vi "Speciality IO Channel Names.vi"(8 "error in (no error)":errorcluster, 10 "channel in":T1, 11 "FPGA Addon ref in":T3 format="%.0x") -> (0 "error out":errorcluster, 2 "channel names out":string[](array[string]), 3 "FPGA Addon ref out":T3 format="%.0x")   [LabVIEW 2026, in "FPGA Addon Bitfile Reload Unit Tests.lvclass"]
uses:
  FPGA Addon Bitfile Reload Unit Tests.lvclass
  <vilib>/NI VeriStand/Custom Device API/Custom Device API.lvlib
  <vilib>/NI VeriStand/Custom Device Tools/Custom Device Utility Library/Custom Device Utility Library.lvlib
  <vilib>/NI VeriStand/Custom Device Tools/Custom Device Utility Library/NI VeriStand - Search for Item by Name.vi
  <vilib>/NI VeriStand/Custom Device API/Custom Device Item Ref.ctl
  APIs/Scripting API/TypeDefs/Output Scalar Data.ctl
  APIs/Scripting API/Scripting API.lvlib
  Addon/Addon Shared/Types/FPGA Addon Data Type.ctl
  Addon/Addon Shared/FPGA Addon Shared.lvlib
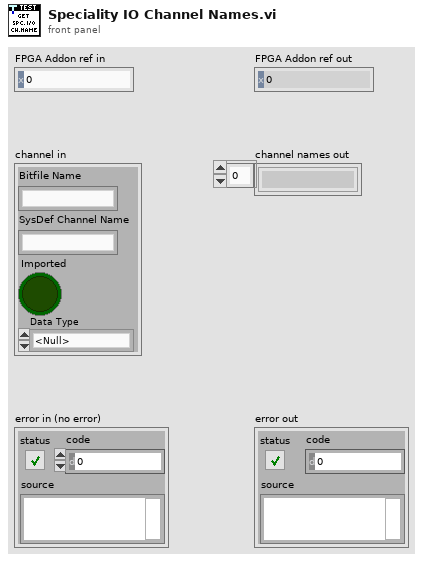
[diagram p1: front panel]
types:
  T1 = typedef "Scripting API.lvlib/Output Scalar Data.ctl" = cluster{"Bitfile Name":string, "SysDef Channel Name":string, "Imported":bool, "Data Type":T2}
  T2 = typedef "FPGA Addon Shared.lvlib/FPGA Addon Data Type.ctl" = enum8{"<Null>", "I8", "I16", "I32", "I64", "U8", "U16", "U32", "U64", "SGL", "Boolean", "Analog PWM In Settings", "Analog PWM In", "Digital PWM In Settings", "Digital PWM In", "Digital PWM Out", "Sine Out", "FXP", "FXP+/-24.5", "FXP+/-16.5", "FXP+/-32.8", "FXP+/-64.32", "FXP+/-16.7", "FXP+/-20.5", "FXP+/-27.5", "FXP+/-32.16", "FXP+16.3", "FXP+18.3", "Digital Static In", "Digital Static Out", "Digital Static In Settings", "Digital WSS Out", "Quad Encoder Settings", "Quad Encoder In", "Group"}
  T3 = typedef "Custom Device API.lvlib/Custom Device Item Ref.ctl" = u64
  T4 = typedef "Custom Device API.lvlib/Custom Device Item Info.ctl" = cluster{"Name":string, "Is Channel":bool, "GUID":string, "Is Waveform":bool}
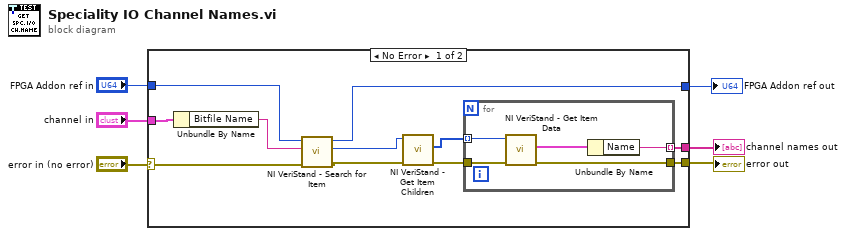
[diagram p0: block diagram]
diagram:
  n1 = case shown="No Error" "error in (no error)" {
    selector: "error in (no error)" -> [w7 w24]
    tunnel: [w15 _] -> w6
    tunnel: [w14 w24] -> w5
    tunnel: "channel in" -> [w13 _]
    tunnel: "FPGA Addon ref in" -> [w12 w23]
    tunnel: [w10 w23] -> w2
    frame No Error {
      n2 = Unbundle By Name(w13) -> ("Bitfile Name"=w11:string)
      n3 = call-poly <vilib>:"NI VeriStand - Search for Item.vi"("error in"=w7, "Item Name"=w11, "Section Ref in"=w12) -> ("error out"=w9:errorcluster, "Item Ref"=w8:T3, "Section Ref out"=w10:T3)  [unwired: 5 in, 1 out]
      n4 = call <vilib>:"NI VeriStand - Get Item Children.vi"("error in (no error)"=w9, "Item Ref in"=w8) -> ("error out"=w17:errorcluster, "Child Refs"=w16:T3[])  [unwired: 6 in, 2 out]
      n5 = for {
        tunnel: w17 -> [w22]
        tunnel: w16 -> [w21] mode=indexing
        tunnel: [w19] -> w15 mode=indexing
        tunnel: [w18] -> w14
        n6 = call <vilib>:"NI VeriStand - Get Item Data.vi"("error in (no error)"=w22, "Item Ref in"=w21) -> ("error out"=w18:errorcluster, "Item Info"=w20:T4)  [unwired: 6 in, 2 out]
        n7 = Unbundle By Name(w20) -> ("Name"=w19:string)
      }
    }
    frame Error {
    }
  }
  "FPGA Addon ref out" <- w2
  "channel names out" <- w6
  "error out" <- w5
